vi "szybka_obwiednia_test.vi"() -> ()   [LabVIEW 2013]
panel:
  in  "Probki do usr":i32
  in  "#Cores (1)":i32=1
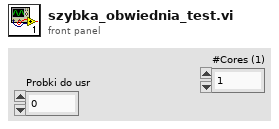
[diagram p1: front panel]
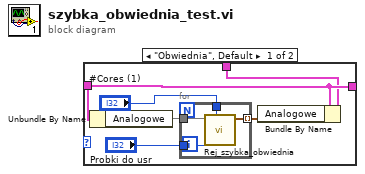
[diagram p0: block diagram]
diagram:
  n1 = case shown="\"Obwiednia\", Default" {
    selector: _ -> [_ _]
    tunnel: _ -> [w3 w11]
    tunnel: [w2 w11] -> _
    tunnel: [w3 w11] -> _
    frame "Obwiednia", Default {
      n2 = Unbundle By Name(w3) -> ("Analogowe"=w6)
      n3 = for {
        tunnel: w6 -> [w10]
        tunnel: [w9] -> w5 mode=indexing
        tunnel: "Probki do usr" -> [w8]
        tunnel: "#Cores (1)" -> [w7]
        n4 = call "Rej_szybka_obwiednia.vi"("Liczba probek (200)"=w8, "#Cores (1)"=w7, "Wfm in"=w10) -> ("Wfm max out"=w9:waveform(dbl))  [unwired: 6 in, 2 out]
      }
      n5 = Bundle By Name(cluster=w3, "Analogowe"=w5) -> (w2:cluster{})
    }
    frame "Migawka" {
    }
  }
